vi "createBroadcastFreezeSensorValuesFrame.vi"(0 "FAILC in":refnum<class "FAILC.lvclass">, 5 "WaitForTrigger":bool, 7 "TriggerIRQ":bool, 9 "BroadcastCounter":u8, 11 "error in (no error)":errorcluster) -> (4 "FAILC out":refnum<class "FAILC.lvclass">, 6 "TxFrame":T1 {"Data" format="%02x"}, 15 "error out":errorcluster)   [LabVIEW 2016, in "RTFAILC.lvlib" / "FAILC.lvclass"]
uses:
  FAILC.lvclass
  Common_RT_Modbus/DataTypes/TxFrame.ctl
  Common_RT_Modbus/DynamicFrameBuilder/DynamicFrameBuilder.lvclass
  FAILC.lvclass/FAILC.ctl
  Common_RT_Modbus/RTModbus.lvlib
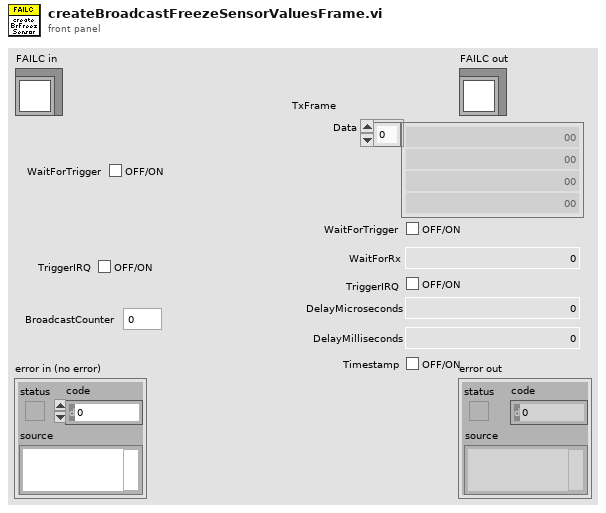
[diagram p1: front panel]
types:
  T1 = typedef "RTModbus.lvlib/TxFrame.ctl" = cluster{"Data":u8[], "WaitForTrigger":bool, "WaitForRx":u16, "TriggerIRQ":bool, "DelayMicroseconds":u16, "DelayMilliseconds":u16, "Timestamp":bool}
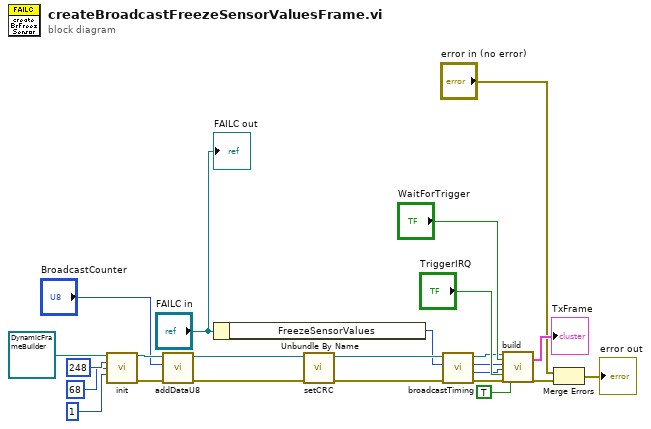
[diagram p0: block diagram]
diagram:
  n1 = call "init.vi"("DynamicFrameBuilder in"=refnum<class "DynamicFrameBuilder.lvclass"> refnum ("RTModbus.lvlib:DynamicFrameBuilder.lvclass"), "Address"=u8 248, "Function"=u8 68, "DataSize"=1) -> ("DynamicFrameBuilder out"=w13:refnum<class "DynamicFrameBuilder.lvclass">, "error out"=w10:errorcluster)  [unwired: 10 in]
  n2 = call "addDataU8.vi"("error in (no error)"=w10, "Data"="BroadcastCounter", "DynamicFrameBuilder in"=w13) -> ("error out"=w9:errorcluster, "DynamicFrameBuilder out"=w12:refnum<class "DynamicFrameBuilder.lvclass">)  [unwired: 7 in]
  n3 = Unbundle By Name("FAILC in") -> ("FreezeSensorValues"=w7:u32)
  n4 = call "setCRC.vi"("error in (no error)"=w9, "DynamicFrameBuilder in"=w12) -> ("error out"=w6:errorcluster, "DynamicFrameBuilder out"=w8:refnum<class "DynamicFrameBuilder.lvclass">)  [unwired: 8 in]
  n5 = call "broadcastTiming.vi"("error in (no error)"=w6, "Latency in"=w7, "DynamicFrameBuilder in"=w8) -> ("error out"=w5:errorcluster, "WaitForRxTimeout"=w2:u16, "Latency out"=w3:u32, "DynamicFrameBuilder out"=w4:refnum<class "DynamicFrameBuilder.lvclass">)  [unwired: 5 in]
  n6 = call "build.vi"("DynamicFrameBuilder in"=w4, "WaitForTrigger"="WaitForTrigger", "Latency"=w3, "WaitForRxTimeout"=w2, "TriggerIRQ"="TriggerIRQ", "error in (no error)"=w5, "Timestamp"=TRUE) -> ("TxFrame"=→"TxFrame":T1, "error out"=w17:errorcluster)  [unwired: 10 in, 1 out]
  n7 = Merge Errors("error in (no error)", w17) -> (→"error out":errorcluster)
  "FAILC out" <- "FAILC in"
